vi "Charger_Monitor Cleanup.vi"(5 "Status Refnum":T1, 6 "error in":errorcluster, 7 "semaphore":T2) -> (0 "error out":errorcluster, 1 "semaphore out":T2)   [LabVIEW 2020]
uses:
  Charger_Status Refnum.ctl
  Drivers/Charger Test Set/Charger_Input Control.ctl
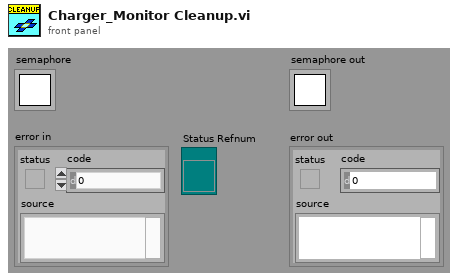
[diagram p1: front panel]
types:
  T1 = typedef "Charger_Status Refnum.ctl" = refnum<vi>
  T2 = typedef "Semaphore RefNum" = refnum<k1>
  T3 = typedef "Charger_Input Control.ctl" = cluster{"address":refnum<visa-resource-name>, "position":i32, "setpoint":dbl}
  T4 = typedef "MICS_Input Control.ctl" = cluster{"address":refnum<visa-resource-name>, "chan":u16, "ID":u32}
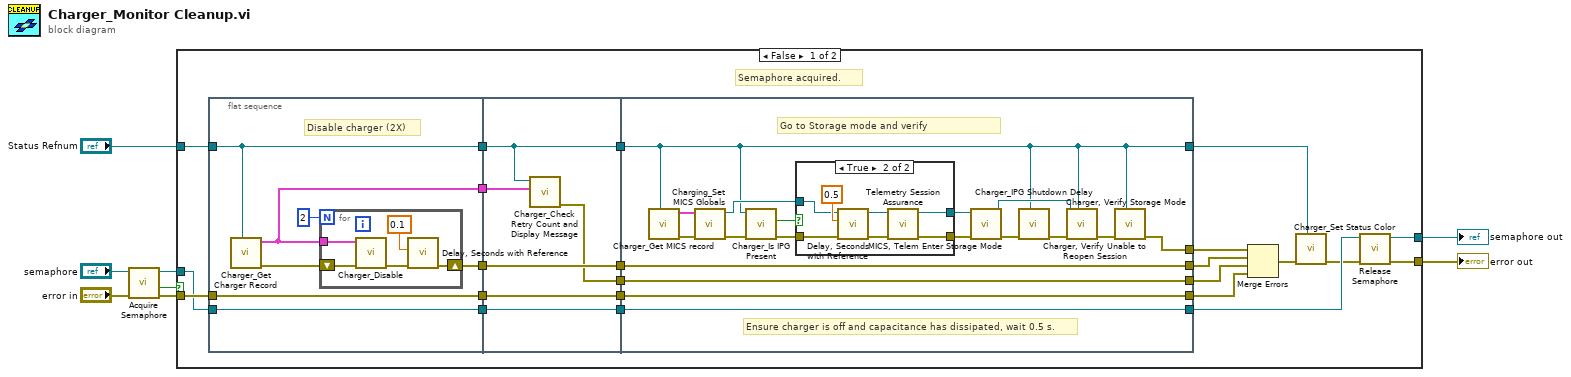
[diagram p0: block diagram]
diagram:
  n1 = call <vilib>:"Acquire Semaphore.vi"("error in (no error)"="error in", "semaphore"="semaphore") -> ("error out"=w2:errorcluster, "timed out"=w3:bool, "semaphore out"=w4:T2)  [unwired: 3 in]
  n2 = case shown="False" w3 {
    tunnel: w2 -> [w25 w77]
    tunnel: [w30 w77] -> w7
    tunnel: w4 -> [w24 w78]
    tunnel: [w31 w78] -> w6
    tunnel: "Status Refnum" -> [w28 _]
    frame False {
      # "Semaphore acquired."
      n3 = flat-sequence {
        tunnel: w28 -> [w36]
        tunnel: w24 -> [w38]
        tunnel: [w38] -> w20
        tunnel: [w36] -> w18
        tunnel: [w35] -> w16
        tunnel: w25 -> [w34]
        tunnel: [w34] -> w14
        tunnel: [w32] -> w12
        tunnel: w20 -> [w49]
        tunnel: [w49] -> w19
        tunnel: w18 -> [w45]
        tunnel: [w45] -> w17
        tunnel: w16 -> [w48]
        tunnel: [w48] -> w15
        tunnel: w14 -> [w47]
        tunnel: [w47] -> w13
        tunnel: w12 -> [w46]
        tunnel: [w44] -> w11
        tunnel: w19 -> [w67]
        tunnel: w17 -> [w52]
        tunnel: [w67] -> w29
        tunnel: [w58] -> w27
        tunnel: [w61] -> w26
        tunnel: w15 -> [w61]
        tunnel: w13 -> [w60]
        tunnel: [w60] -> w10
        tunnel: [w52] -> w21
        tunnel: w11 -> [w50]
        tunnel: [w50] -> w9
        frame #0 {
          # "Disable charger (2X)"
          n4 = call "Charger_Get Charger Record.vi"("Status Refnum"=w36) -> ("error out"=w37:errorcluster, "Charger Inputs"=w32:T3)  [unwired: 4 in, 3 out]
          n5 = for {
            N: 2 -> [_]
            tunnel: w32 -> [w43]
            shift-right: [w39] -> w35
            shift-left: w37 -> [w42]
            n6 = call "Charger_Disable.vi"("error in"=w42, "Charger"=w43) -> ("error out"=w40:errorcluster)  [unwired: 7 in]
            n7 = call "Delay, Seconds with Reference.vi"("error in"=w40, "delay"=dbl[unit] 0.1) -> ("error out"=w39:errorcluster)  [unwired: 4 in, 2 out]
          }
        }
        frame #1 {
          n8 = call "Charger_Check Retry Count and Display Message.vi"("Charger Inputs"=w46, "Status Refnum"=w45) -> ("error out"=w44:errorcluster)  [unwired: 9 in]
        }
        frame #2 {
          # "Ensure charger is off and capacitance has dissipated, wait 0.5 s."
          # "Go to Storage mode and verify"
          n9 = call "Charger_Get MICS record.vi"("Status Refnum"=w52) -> ("error out"=w65:errorcluster, "MICS Inputs"=w64:T4)  [unwired: 4 in, 3 out]
          n10 = call "Charging_Set MICS Globals.vi"("error in"=w65, "MICS inputs"=w64) -> ("error out"=w55:errorcluster, "address"=w53:refnum<visa-resource-name>)  [unwired: 4 in]
          n11 = call "Charger_Is IPG Present.vi"("error in"=w55, "Status Refnum"=w52) -> ("error out"=w54:errorcluster, "IPG Present?"=w51:bool)  [unwired: 7 in, 1 out]
          n12 = case shown="True" w51 {
            tunnel: [w69 w73] -> w57
            tunnel: [w68 w71] -> w56
            tunnel: w54 -> [w68 w75]
            tunnel: w53 -> [w69 w74]
            frame False {
            }
            frame True {
              n13 = call "Delay, Seconds with Reference.vi"("error in"=w75, "delay"=dbl[unit] 0.5, "VISA resource"=w74) -> ("error out"=w72:errorcluster, "VISA resource dup"=w70:refnum<visa-resource-name>)  [unwired: 3 in, 1 out]
              n14 = call "Telemetry Session Assurance.vi"("error in"=w72, "MICS Dongle Address"=w70) -> ("error out"=w71:errorcluster, "MICS Dongle Address dup"=w73:refnum<visa-resource-name>)  [unwired: 8 in]
            }
          }
          n15 = call "MICS, Telem Enter Storage Mode.vi"("error in"=w56, "VISA resource"=w57) -> ("error out"=w63:errorcluster, "VISA resource dup"=w66:refnum<visa-resource-name>)  [unwired: 8 in]
          n16 = call "Charger_IPG Shutdown Delay.vi"("Status Refnum"=w52, "error in"=w63) -> ("error out"=w62:errorcluster)  [unwired: 7 in]
          n17 = call "Charger, Verify Storage Mode.vi"("error in"=w62, "VISA resource"=w66, "Status Refnum"=w52) -> ("error out"=w59:errorcluster)  [unwired: 6 in, 1 out]
          n18 = call "Charger, Verify Unable to Reopen Session.vi"("error in"=w59, "Status Refnum"=w52) -> ("error out"=w58:errorcluster)  [unwired: 8 in]
        }
      }
      n19 = Merge Errors(w27, w26, w9, w10) -> (w23:errorcluster)
      n20 = call "Charger_Set Status Color.vi"("error in"=w23, "Status Refnum"=w21) -> ("error out"=w22:errorcluster)  [unwired: 8 in]
      n21 = call <vilib>:"Release Semaphore.vi"("error in (no error)"=w22, "semaphore"=w29) -> ("error out"=w30:errorcluster, "semaphore out"=w31:T2)  [unwired: 4 in]
    }
    frame True {
      # "Semaphore timed out."
    }
  }
  "error out" <- w7
  "semaphore out" <- w6
